vi "Array_dualslicer.vi"(0 "X array":dbl[](array[numeric]), 1 "Y array":dbl[](array[numeric]), 2 "Slicing array":bool[](array[boolean]), 3 "error in":errorcluster) -> (4 "Y Output array":dbl[][](array[numeric]), 5 "error out":errorcluster, 6 "Indices":i32[](array[numeric]), 7 "X Output array":dbl[][](array[numeric]), 8 "Lengths":i32[](array[numeric]), 9 "Output cluster":cluster{dbl[], dbl[]}[](array[cluster]))   [LabVIEW 2016]
doc: "Slice the input array before every indices where slicing array is True and output a 2D array containing all these subarrays in order"
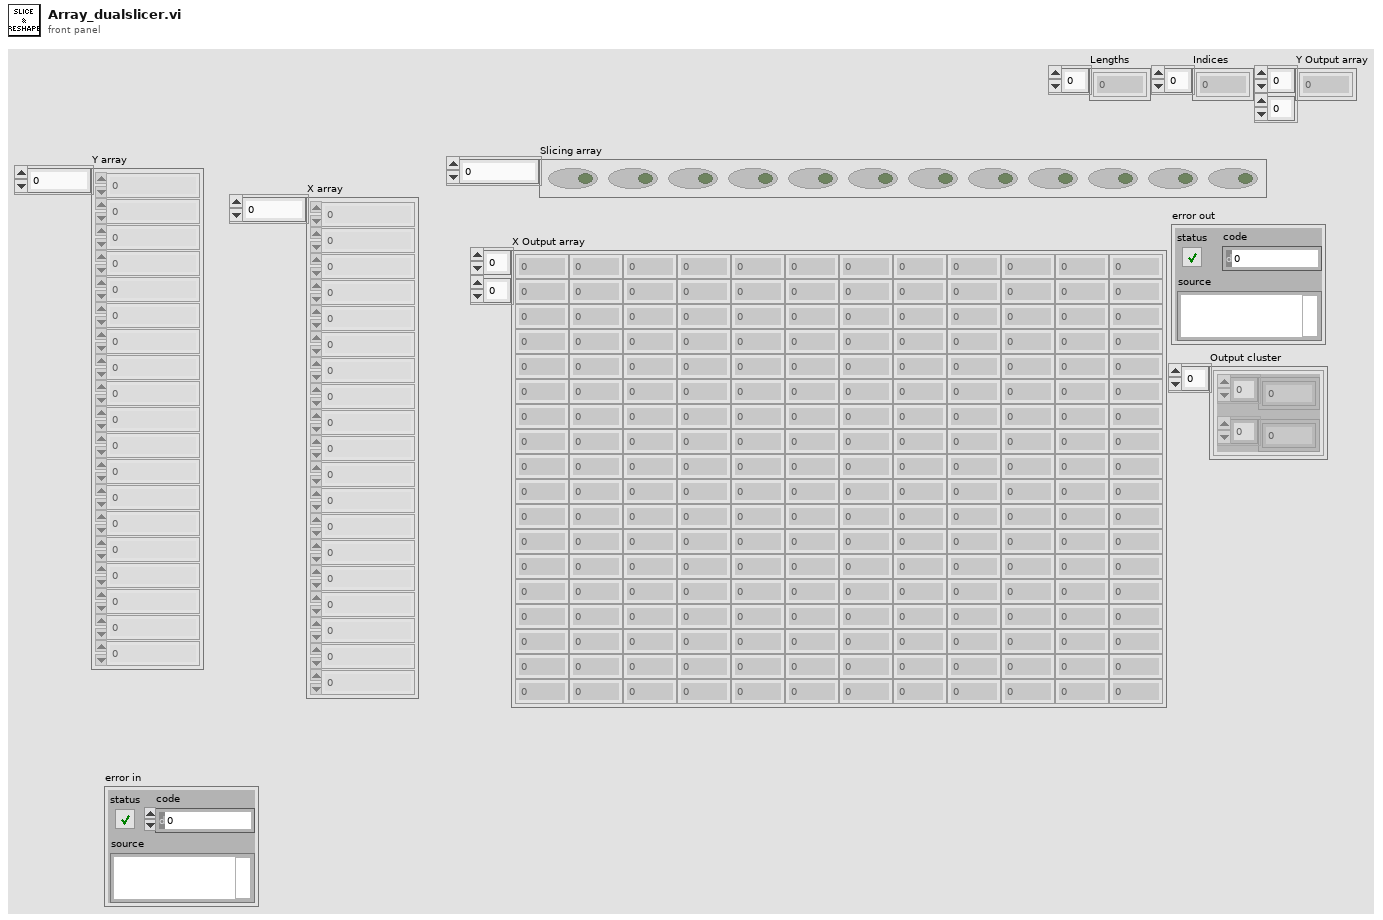
[diagram p1: front panel]
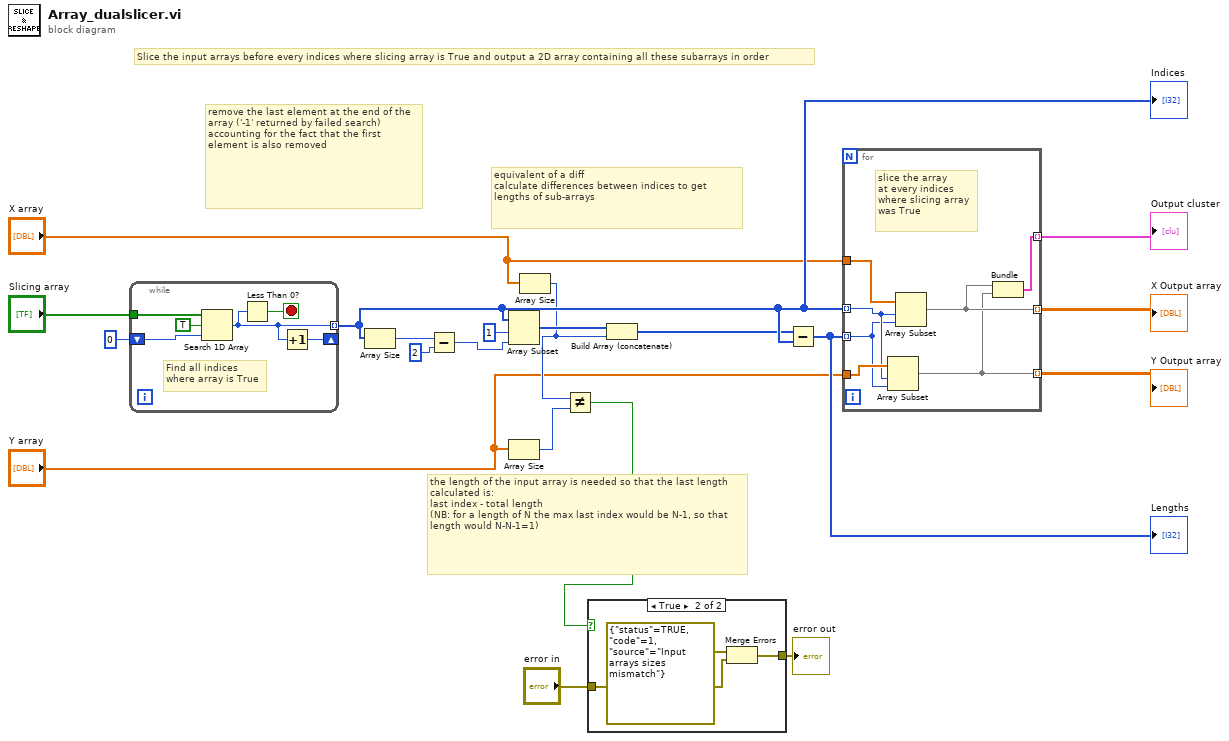
[diagram p0: block diagram]
diagram:
  # "Slice the input arrays before every indices where slicing array is True and output a 2D array containing all these subarrays in order"
  # "the length of the input array is needed so that the last length calculated is: \nlast index - total length\n(NB: for a length of N the max last index would be N-1, so that length would N-N-1=1)"
  # "remove the last element at the end of the array ('-1' returned by failed search) accounting for the fact that the first element is also removed"
  # "equivalent of a diff\ncalculate differences between indices to get lengths of sub-arrays"
  n1 = while {
    tunnel: "Slicing array" -> [w26]
    shift-right: [w23] -> _
    shift-left: 0 -> [w21]
    tunnel: [w22] -> w16 mode=indexing
    stop <- w24 stop-if-true
    # "Find all indices\nwhere array is True"
    n2 = Search 1D Array(1D array=w26, element=TRUE, start index (0)=w21) -> (index of element=w22:i32)
    n3 = Less Than 0?(x=w22) -> (x < 0?=w24:bool)
    n4 = Increment(x=w22) -> (x+1=w23:i32)
  }
  "Indices" <- w16
  n5 = Array Size(array=w16) -> (size(s)=w11:i32)
  n6 = Subtract(x=w11, y=2) -> (x-y=w14:i32)
  n7 = Array Subset(array=w16, index=1, length=w14) -> (w18:i32[])
  n8 = Array Size(array="Y array") -> (size(s)=w8:i32)
  n9 = Array Size(array="X array") -> (size(s)=w7:i32)
  n10 = Not Equal?(x=w7, y=w8) -> (x != y?=w4:bool)
  n11 = case shown="True" w4 {
    tunnel: "error in" -> [w27 w28]
    tunnel: [w27 w30] -> w5
    frame False {
    }
    frame True {
      n12 = Merge Errors(errorcluster {"status"=TRUE, "code"=1, "source"="Input arrays sizes mismatch"} ("error constant"), w28) -> (w30:errorcluster)
    }
  }
  "error out" <- w5
  n13 = Build Array (concatenate)(w18, w7) -> (w15:i32[])
  n14 = Subtract(x=w15, y=w16) -> (x-y=w17:i32[])
  "Lengths" <- w17
  n15 = for {
    tunnel: w16 -> [w35] mode=indexing
    tunnel: w17 -> [w34] mode=indexing
    tunnel: "X array" -> [w37]
    tunnel: [w33] -> w9 mode=indexing
    tunnel: "Y array" -> [w36]
    tunnel: [w32] -> w2 mode=indexing
    tunnel: [w31] -> w1 mode=indexing
    # "slice the array\nat every indices\nwhere slicing array\nwas True"
    n16 = Array Subset(array=w36, index=w35, length=w34) -> (w32:dbl[])
    n17 = Array Subset(array=w37, index=w35, length=w34) -> (w33:dbl[])
    n18 = Bundle(w33, w32) -> (w31:cluster{dbl[], dbl[]})  [unwired: 1 in]
  }
  "X Output array" <- w9
  "Y Output array" <- w2
  "Output cluster" <- w1
